vi "Open Sample Container Connections.vi"(8 "error in (no error)":errorcluster, 11 "Syringe in":refnum<class "Syringe Line.lvclass">) -> (0 "error out":errorcluster, 3 "Syringe out":refnum<class "Syringe Line.lvclass">)   [LabVIEW 2015, in "cRIO-Carbondioxide.lvlib" / "CO2-Actor.lvlib" / "Syringe Line.lvclass"]
uses:
  Syringe Line.lvclass
  Syringe Line.lvclass/Syringe Line.ctl
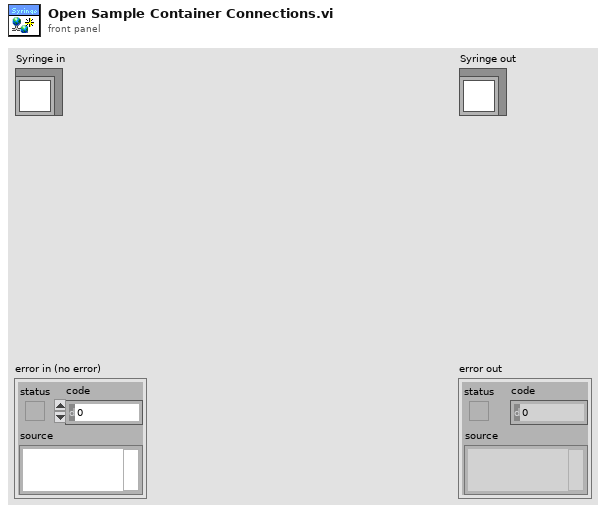
[diagram p1: front panel]
types:
  T1 = typedef "Sample Container.ctl" = cluster{"Sample In":refnum<k21>, "Sample Name":refnum<k21>, "Ti Cathode":refnum<k21>, "SampleQ":refnum<queue>}
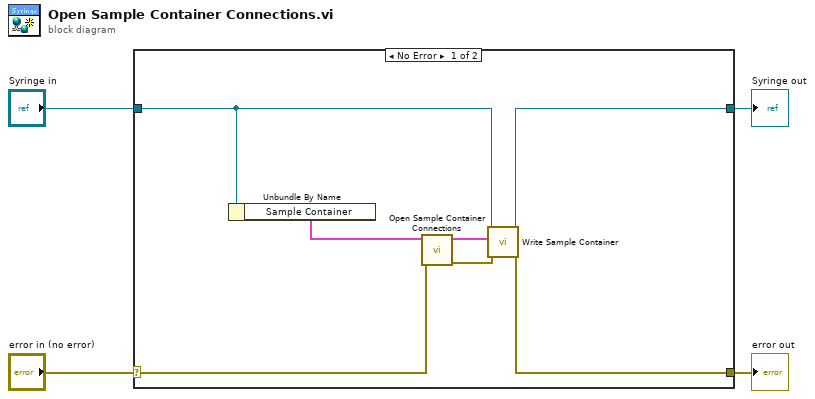
[diagram p0: block diagram]
diagram:
  n1 = case shown="No Error" "error in (no error)" {
    selector: "error in (no error)" -> [w7 w13]
    tunnel: [w8 w13] -> w3
    tunnel: [w10 w12] -> w1
    tunnel: "Syringe in" -> [w6 w12]
    frame No Error {
      n2 = Unbundle By Name(w6) -> ("Sample Container"=w5:T1)
      n3 = call "Open Sample Container Connections.vi"("error in (no error)"=w7, "Container in"=w5) -> ("error out"=w9:errorcluster, "Container out"=w11:T1)  [unwired: 8 in]
      n4 = call "Write Sample Container.vi"("error in (no error)"=w9, "Sample Container"=w11, "Syringe in"=w6) -> ("error out"=w8:errorcluster, "Syringe out"=w10:refnum<class "Syringe Line.lvclass">)  [unwired: 7 in]
    }
    frame Error {
    }
  }
  "error out" <- w3
  "Syringe out" <- w1
